vi "Async.Engine.Write Data to HW.vi"(8 "error in":errorcluster, 11 "VS Plugin Inline Async API in":refnum<class "VS Plugin Inline Async API.lvclass">) -> (0 "error out":errorcluster, 3 "VS Plugin Inline Async API out":refnum<class "VS Plugin Inline Async API.lvclass">)   [LabVIEW 2024, in "VS Plugin Inline Async API.lvlib" / "VS Plugin Inline Async API.lvclass"]
uses:
  VS Plugin Inline Async API.lvclass
  VS Plugin Inline Async API.lvclass/VS Plugin Inline Async API.ctl
  Plugin Data Access/Plugin Data Access.lvclass
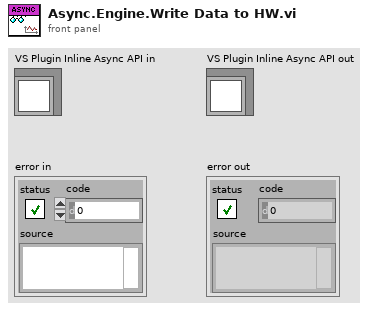
[diagram p1: front panel]
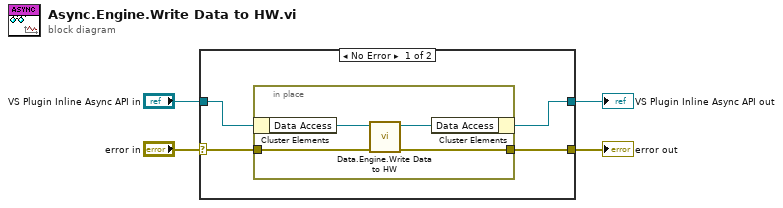
[diagram p0: block diagram]
diagram:
  n1 = case shown="No Error" "error in" {
    selector: "error in" -> [w8 w14]
    tunnel: [w7 w14] -> w3
    tunnel: [w5 w13] -> w1
    tunnel: "VS Plugin Inline Async API in" -> [w6 w13]
    frame No Error {
      n2 = in-place {
        in-place-border: w8 -> [w12]
        in-place-border: [w11] -> w7
        n3 = in-place-cluster #1(w6) -> ("Data Access"=w10:refnum<class "Plugin Data Access.lvclass">)
        n4 = call "Data.Engine.Write Data to HW.vi"("error in"=w12, "Plugin Data Access in"=w10) -> ("error out"=w11:errorcluster, "Plugin Data Access out"=w9:refnum<class "Plugin Data Access.lvclass">)  [unwired: 8 in]
        n5 = in-place-cluster #1("Data Access"=w9) -> (w5:refnum<class "VS Plugin Inline Async API.lvclass">)
      }
    }
    frame Error {
    }
  }
  "error out" <- w3
  "VS Plugin Inline Async API out" <- w1
